vi "Hardware Discovery.vi"() -> ()   [LabVIEW 2020]
uses:
  subVIs/TypeDefs/rad_State Data.ctl
  subVIs/Targets/TypeDefs/rad_Targets Settings.ctl
  support/SubVIs/Target Information.ctl
  subVIs/Targets/TypeDefs/rad_Target Network Settings.ctl
  support/Controls/Discovery Settings.ctl
  support/Controls/Discovery Method Enum.ctl
  support/Controls/Important Paths.ctl
  subVIs/Util/Controls/Exit Button.ctl
  subVIs/Util/Controls/Refresh Button.ctl
  subVIs/Util/Controls/Configure Button.ctl
  subVIs/Util/Controls/Select All Button.ctl
  subVIs/Util/Controls/Add Target Button.ctl
  support/Controls/SetUp Btn.ctl
  subVIs/Util/FP Control/FP Control Functions.ctl
  <vilib>/Utility/miscctls.llb/LVRowAndColumnUnsignedTypeDef.ctl
  support/Message Queue/Enqueue Message (Single).vi
  <vilib>/nisyscfg/Close (System).vi
  support/Message Queue/Message Queue.lvlib
  <vilib>/nisyscfg/nisyscfg.lvlib
  <resource>/objmgr/nisysapi.rc
panel:
  in  "Set Up Target":T1
  in  "Exit":T2
  in  "Target List":i32[](listbox)=[0]
  in  "Refresh Targets":T3
  in  "Targets Settings":bool
  in  "Add Target":T4
  in  "Select All":T5
  in  "Configure Targets":T6
  in  "App Data":T7 {"Targets Information"."Primary NIC"."IP Address Request Mode" items=["Static"=1, "DHCP/Link-Local"=2, "Link-Local Only"=4, "DHCP Only"=8]}
  # "Detected Targets"
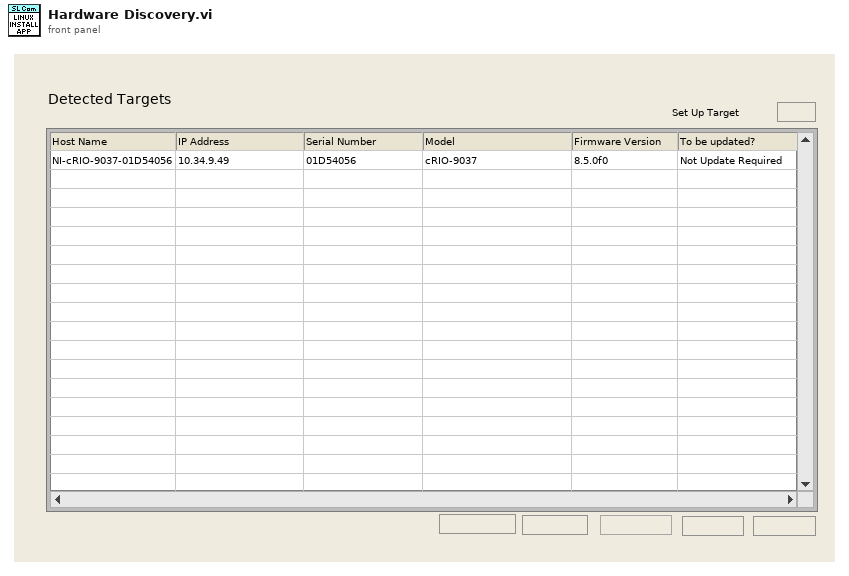
[diagram p1: front panel]
types:
  T1 = typedef "SetUp Btn.ctl" = bool
  T2 = typedef "Exit Button.ctl" = bool
  T3 = typedef "Refresh Button.ctl" = bool
  T4 = typedef "Add Target Button.ctl" = bool
  T5 = typedef "Select All Button.ctl" = bool
  T6 = typedef "Configure Button.ctl" = bool
  T7 = typedef "rad_State Data.ctl" = cluster{"Targets Settings":T8, "Targets Information":T9[], "Filtered Targets":i32[], "AppMode":string, "Configuration File Path":path, "Permissions":cluster{"Retrieve AppImgs":bool}, "User Added Targets":string[], "Discovery":T11, "Important Paths":T13}
  T8 = typedef "rad_Targets Settings.ctl" = cluster{"Target Types":string[], "Reduce Discovery Timeout":bool}
  T9 = typedef "Target Information.ctl" = cluster{"Hostname":string, "Serial number":string, "Product name":string, "Product code":i32, "System status":string, "Credential type":enum16{"None/Unlocked", "FTP Password", "NIAuth Credentials"}, "User added?":bool, "Primary NIC":T10}
  T10 = typedef "rad_Target Network Settings.ctl" = cluster{"MAC address":string, "IP Address Request Mode":i32, "IP address":string, "Subnet mask":string, "Gateway":string, "DNS server":string}
  T11 = typedef "Discovery Settings.ctl" = cluster{"Method":T12, "NotAsk":bool, "IPsFilePath":path}
  T12 = typedef "Discovery Method Enum.ctl" = enum32{"USB", "IPsFile", "AutoAll", "NotDiscover"}
  T13 = typedef "Important Paths.ctl" = cluster{"Linux Base Image":path, "Firmware Locations":path, "System Configuration Version":string}
  T14 = typedef "LVPoint32TypeDef.ctl" = cluster{"Horizontal":i32, "Vertical":i32}
  T15 = typedef "LVRowAndColumnTypeDef.ctl" = cluster{"Row":i32, "Column":i32}
  T16 = typedef "LVRowAndColumnUnsignedTypeDef.ctl" = cluster{"Row":u32, "Column":u32}
  T17 = enum8{"Enabled", "Disabled", "Disabled and Grayed Out"}
  T18 = typedef "FP Control Functions.ctl" = enum16{"Open", "Close", "Bring To Front", "Center"}
  T19 = enum32{"invalid app kind", "Development System", "Run Time System", "Student Edition", "Embedded LabVIEW", "Evaluation", "Custom"}
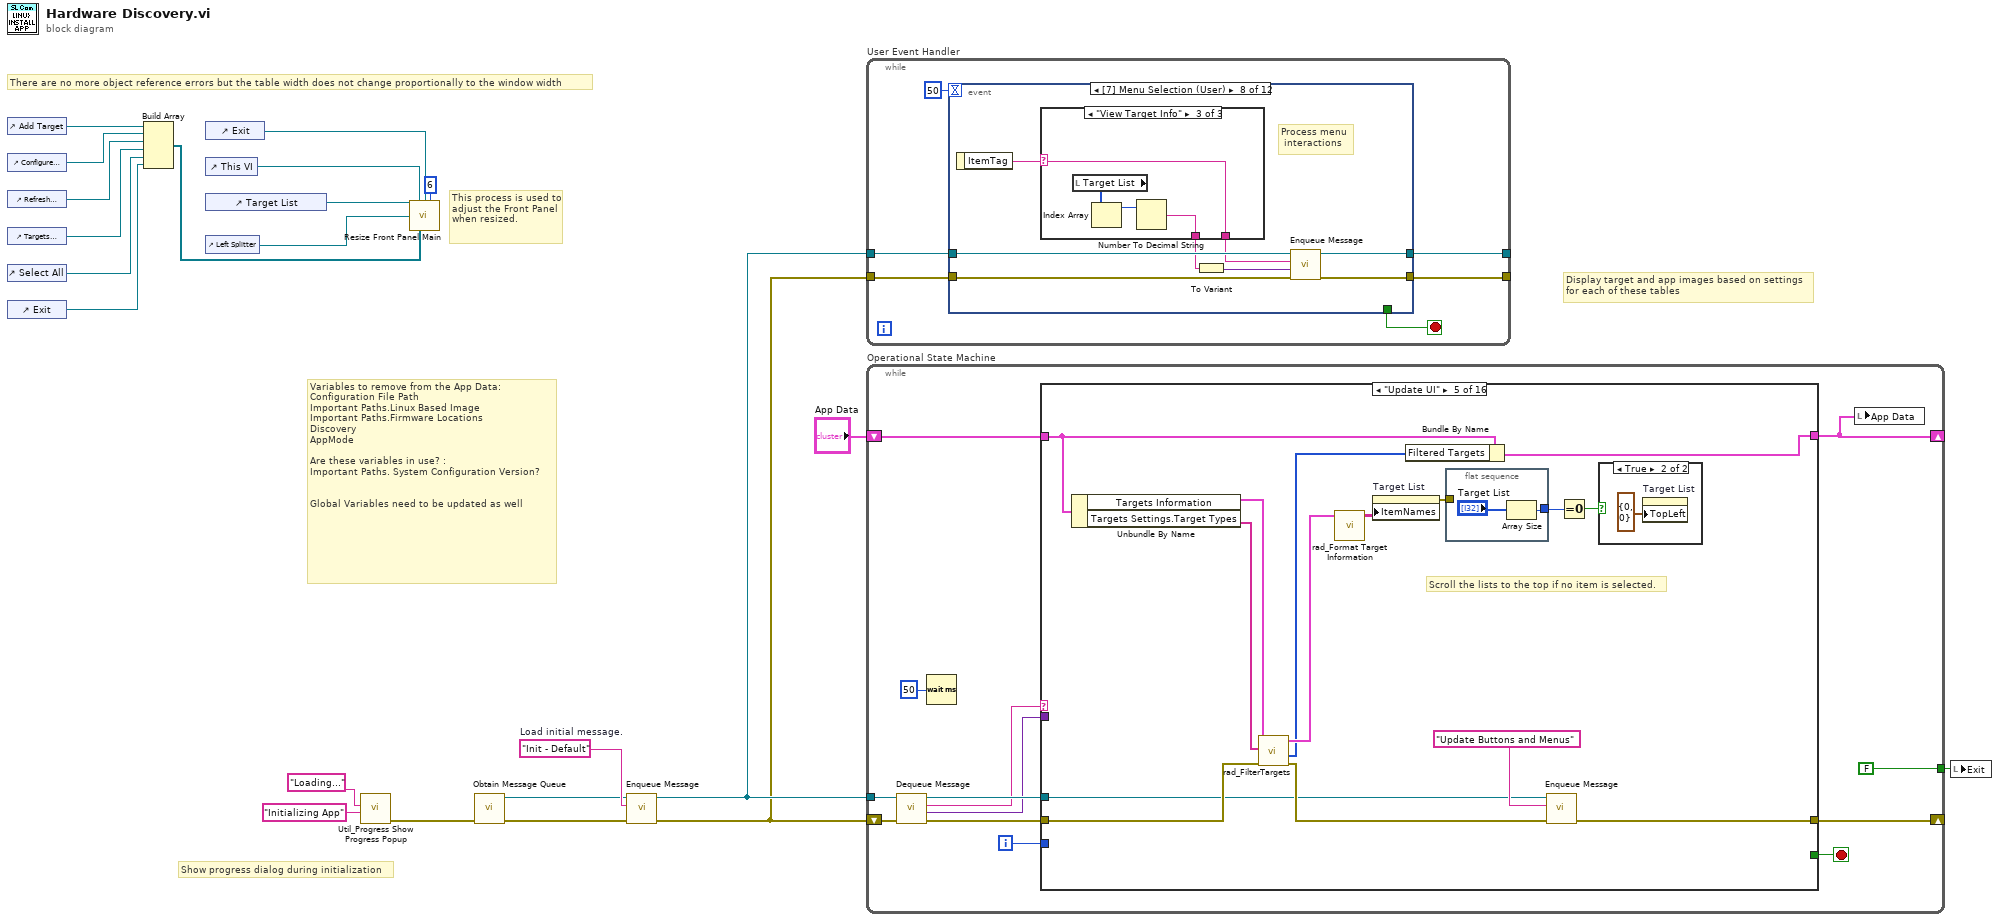
[diagram p0: block diagram]
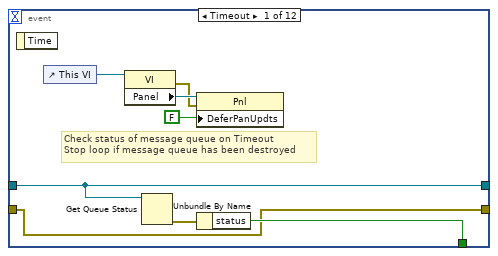
[diagram p2: hidden frame]
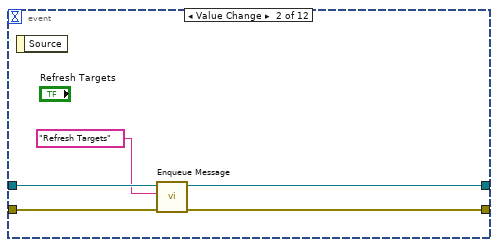
[diagram p3: hidden frame]
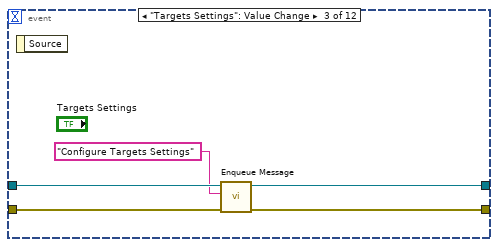
[diagram p4: hidden frame]
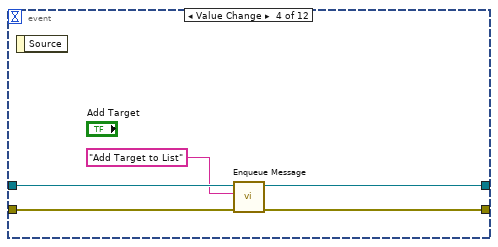
[diagram p5: hidden frame]
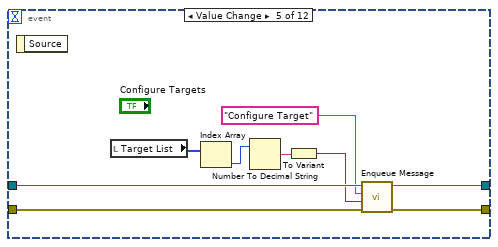
[diagram p6: hidden frame]
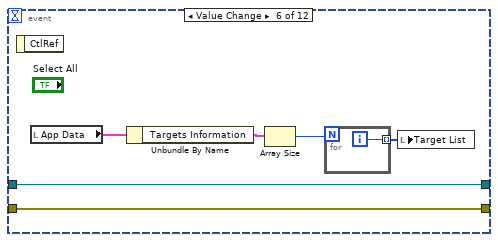
[diagram p7: hidden frame]
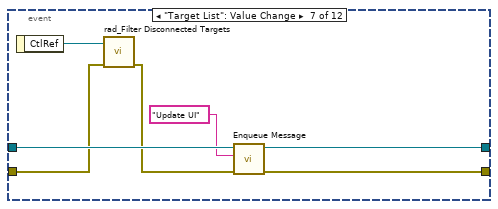
[diagram p8: hidden frame]
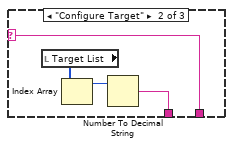
[diagram p10: hidden frame]
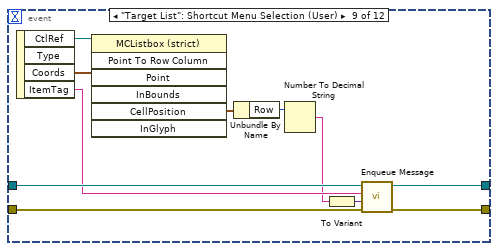
[diagram p11: hidden frame]
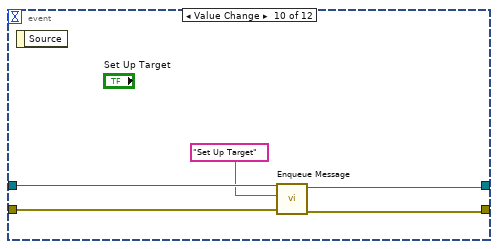
[diagram p12: hidden frame]
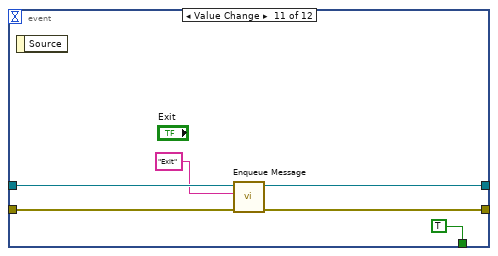
[diagram p13: hidden frame]
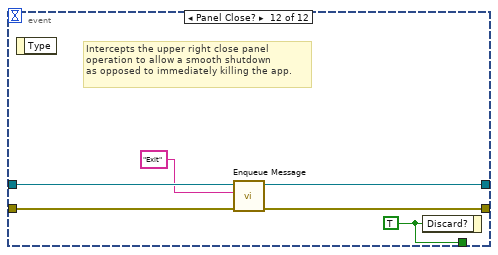
[diagram p14: hidden frame]
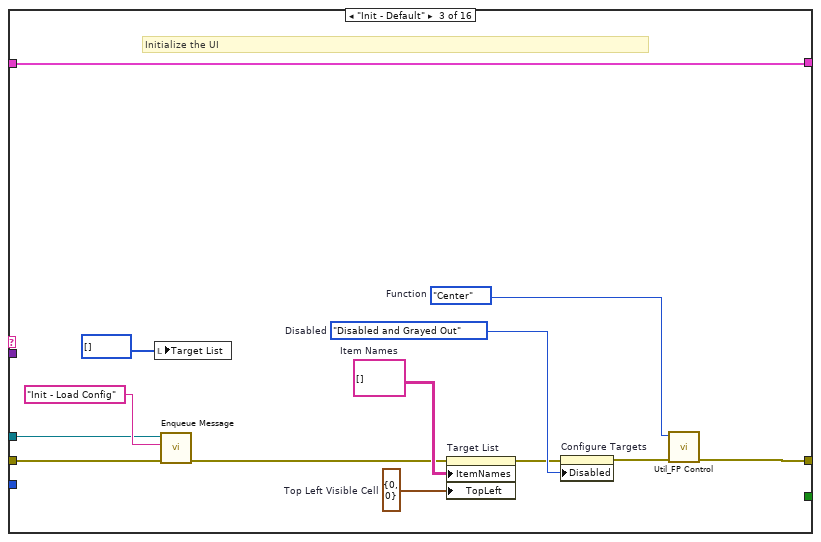
[diagram p17: hidden frame]
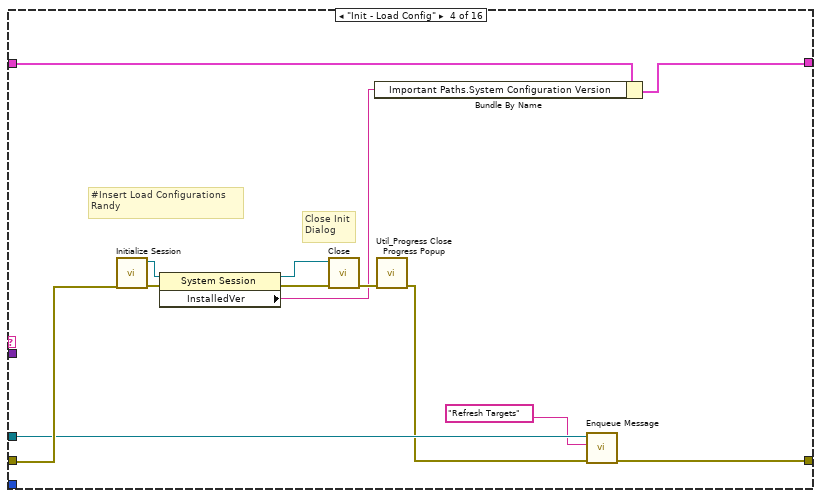
[diagram p18: hidden frame]
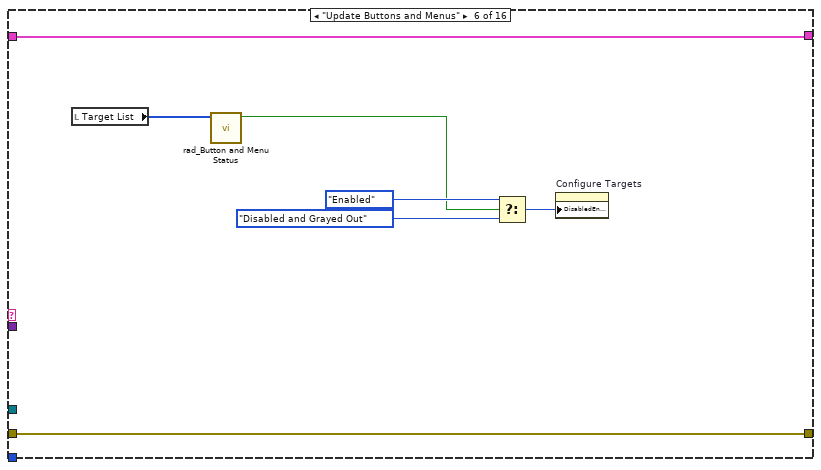
[diagram p20: hidden frame]
diagram:
  w8 = "Init - Default"  # Load initial message.
  # "Variables to remove from the App Data:\nConfiguration File Path\nImportant Paths.Linux Based Image\nImportant Paths.Firmware Locations\nDiscovery\nAppMode\n\nAre these variables in use? :\nImportant Paths. System Configuration Version?\n\n\nGlobal Variables need to be updated as well"
  # "There are no more object reference errors but the table width does not change proportionally to the window width"
  # "Display target and app images based on settings\nfor each of these tables"
  # "Show progress dialog during initialization"
  # "This process is used to adjust the Front Panel when resized."
  n1 = control-ref of="Add Target"() -> (w17:refnum<vi>)
  n2 = control-ref of="Configure Targets"() -> (w16:refnum<vi>)
  n3 = control-ref of="Refresh Targets"() -> (w15:refnum<vi>)
  n4 = control-ref of="Targets Settings"() -> (w14:refnum<vi>)
  n5 = control-ref of="Select All"() -> (w13:refnum<vi>)
  n6 = control-ref of="Exit"() -> (w3:refnum<vi>)
  n7 = Build Array(w17, w16, w15, w14, w13, w3) -> (w12:refnum<vi>[])
  n8 = control-ref of="Exit"() -> (w21:refnum<vi>)
  n9 = control-ref of="This VI"() -> (w20:refnum<vi>)
  n10 = control-ref of="Target List"() -> (w19:refnum<vi>)
  n11 = control-ref of="Left Splitter"() -> (w18:refnum<vi>)
  n12 = call "Util_Progress Show Progress Popup.vi"("Title"="Initializing App", "Message"="Loading...") -> ("error out"=w10:errorcluster)  [unwired: 2 in, 7 out]
  n13 = call "Resize Front Panel Main.vi"("Left Listbox"=w19, "Top Level VI"=w20, "Stop"=w21, "Number of Columns"=6, "Left Splitter"=w18, "Left Pane Items"=w12) -> ()  [unwired: 9 in, 1 out]
  n14 = call "Obtain Message Queue.vi"("error in (no error)"=w10) -> ("error out"=w9:errorcluster, "Message Queue"=w7:refnum<queue>)  [unwired: 9 in]
  n15 = call-poly "Enqueue Message.vi"("error in (no error)"=w9, "Message"=w8, "Message Queue"=w7) -> ("error out"=w5:errorcluster, "dup Message Queue"=w6:refnum<queue>)  [unwired: 7 in]
  n16 = while "User Event Handler" {
    tunnel: w6 -> [w26]
    tunnel: [w25] -> _
    tunnel: w5 -> [w24]
    tunnel: [w23] -> _
    stop <- w27 stop-if-true
    n17 = event shown="[7] Menu Selection (User)" {
      selector: _ -> [_ _ _ _ _ _ _ _ _ _ _ _]
      dyn-events: _ -> [_ _ _ _ _ _ _ _ _ _ _ _]
      timeout: 50 -> [_ _ _ _ _ _ _ _ _ _ _ _]
      tunnel: [w34 _ _ _ _ _ _ _ _ _ TRUE ("Discard?") w119] -> w27
      tunnel: w26 -> [w36 w41 w44 w49 w56 w62 w72 w79 w96 w107 w110 w116]
      tunnel: [w36 w40 w43 w48 w55 w62 w71 w78 w95 w105 w109 w115] -> w25
      tunnel: w24 -> [w29 w39 w46 w51 w58 w61 w68 w81 w98 w106 w112 w118]
      tunnel: [w29 w38 w45 w50 w57 w61 w73 w80 w97 w104 w111 w117] -> w23
      event Timeout {
        # "Check status of message queue on Timeout\nStop loop if message queue has been destroyed"
        n18 = event-data() -> ()  [unwired: 2 out]
        n19 = control-ref of="This VI"() -> (w30:refnum<vi>)
        n20 = property class="VI"(reference=w30) -> (error out=w31:errorcluster, "Panel"=w33:refnum<vi>)  [unwired: 1 in, 1 out]
        n21 = Get Queue Status(queue=w36) -> (error out=w35:errorcluster)  [unwired: 1 in, 8 out]
        n22 = property class="Pnl"(reference=w33, error in=w31, "DeferPanUpdts"=FALSE ("Defer Panel Updates")) -> ()  [unwired: 2 out]
        n23 = Unbundle By Name(w35) -> ("status"=w34:bool)
      }
      event Value Change {
        n24 = event-data() -> ()  [unwired: 2 out]
        n25 = call-poly "Enqueue Message.vi"("error in (no error)"=w39, "Message"="Refresh Targets", "Message Queue"=w41) -> ("error out"=w38:errorcluster, "dup Message Queue"=w40:refnum<queue>)  [unwired: 7 in]
      }
      event "Targets Settings": Value Change {
        n26 = event-data() -> ()  [unwired: 2 out]
        n27 = call-poly "Enqueue Message.vi"("error in (no error)"=w46, "Message"="Configure Targets Settings", "Message Queue"=w44) -> ("error out"=w45:errorcluster, "dup Message Queue"=w43:refnum<queue>)  [unwired: 7 in]
      }
      event Value Change {
        n28 = event-data() -> ()  [unwired: 2 out]
        n29 = call-poly "Enqueue Message.vi"("error in (no error)"=w51, "Message"="Add Target to List" ("Message Name"), "Message Queue"=w49) -> ("error out"=w50:errorcluster, "dup Message Queue"=w48:refnum<queue>)  [unwired: 7 in]
      }
      event Value Change {
        n30 = event-data() -> ()  [unwired: 2 out]
        n31 = local read "Target List"() -> (w59:i32[])
        n32 = Index Array(array=w59) -> (element=w60:i32)  [unwired: 1 in]
        n33 = Number To Decimal String(number=w60) -> (decimal integer string=w54:string)  [unwired: 1 out]
        n34 = To Variant(anything=w54) -> (Variant=w53:variant)
        n35 = call-poly "Enqueue Message.vi"("error in (no error)"=w58, "Message Data"=w53, "Message"="Configure Target", "Message Queue"=w56) -> ("error out"=w57:errorcluster, "dup Message Queue"=w55:refnum<queue>)  [unwired: 6 in]
      }
      event Value Change {
        n36 = event-data() -> ()  [unwired: 2 out]
        n37 = local read "App Data"() -> (w65:T7)
        n38 = Unbundle By Name(w65) -> ("Targets Information"=w64:T9[])
        n39 = Array Size(array=w64) -> (size(s)=w63:i32)
        n40 = for {
          N: w63 -> [_]
          tunnel: [w67] -> w66 mode=indexing
          i -> [w67]
        }
        n41 = local write "Target List"(w66) -> ()
      }
      event "Target List": Value Change {
        n42 = event-data() -> ("CtlRef"=w74:refnum<vi>)  [unwired: 1 out]
        n43 = call "rad_Filter Disconnected Targets.vi"("error in (no error)"=w68, "Target List Ref"=w74) -> ("error out"=w69:errorcluster)  [unwired: 9 in]
        n44 = call-poly "Enqueue Message.vi"("error in (no error)"=w69, "Message"="Update UI", "Message Queue"=w72) -> ("error out"=w73:errorcluster, "dup Message Queue"=w71:refnum<queue>)  [unwired: 7 in]
      }
      event Menu Selection (User) {
        # "Process menu\n interactions"
        n45 = event-data() -> ("ItemTag"=w82:string)  [unwired: 1 out]
        n46 = case shown="\"View Target Info\"" w82 {
          selector: w82 -> [w83 w85 w89]
          tunnel: [w83 w85 w89] -> w77
          tunnel: [_ w84 w88] -> w76
          frame Default {
          }
          frame "Configure Target" {
            n47 = local read "Target List"() -> (w87:i32[])
            n48 = Index Array(array=w87) -> (element=w86:i32)  [unwired: 1 in]
            n49 = Number To Decimal String(number=w86) -> (decimal integer string=w84:string)  [unwired: 1 out]
          }
          frame "View Target Info" {
            n50 = local read "Target List"() -> (w91:i32[])
            n51 = Index Array(array=w91) -> (element=w90:i32)  [unwired: 1 in]
            n52 = Number To Decimal String(number=w90) -> (decimal integer string=w88:string)  [unwired: 1 out]
          }
        }
        n53 = To Variant(anything=w76) -> (Variant=w75:variant)
        n54 = call-poly "Enqueue Message.vi"("error in (no error)"=w81, "Message Data"=w75, "Message"=w77, "Message Queue"=w79) -> ("error out"=w80:errorcluster, "dup Message Queue"=w78:refnum<queue>)  [unwired: 6 in]
      }
      event "Target List": Shortcut Menu Selection (User) {
        n55 = event-data() -> ("CtlRef"=w100:refnum<vi>, "Coords"=w99:T14, "ItemTag"=w94:string)  [unwired: 2 out]
        n56 = invoke class="MCListbox (strict)" method="Point To Row Column"(reference=w100, "Point"=w99) -> ("CellPosition"=w102:T15)  [unwired: 5 in, 6 out]
        n57 = Unbundle By Name(w102) -> ("Row"=w101:i32)
        n58 = Number To Decimal String(number=w101) -> (decimal integer string=w93:string)  [unwired: 1 out]
        n59 = To Variant(anything=w93) -> (Variant=w92:variant)
        n60 = call-poly "Enqueue Message.vi"("error in (no error)"=w98, "Message Data"=w92, "Message"=w94, "Message Queue"=w96) -> ("error out"=w97:errorcluster, "dup Message Queue"=w95:refnum<queue>)  [unwired: 6 in]
      }
      event Value Change {
        n61 = event-data() -> ()  [unwired: 2 out]
        n62 = call-poly "Enqueue Message.vi"("error in (no error)"=w106, "Message"="Set Up Target", "Message Queue"=w107) -> ("error out"=w104:errorcluster, "dup Message Queue"=w105:refnum<queue>)  [unwired: 7 in]
      }
      event Value Change {
        n63 = event-data() -> ()  [unwired: 2 out]
        n64 = call-poly "Enqueue Message.vi"("error in (no error)"=w112, "Message"="Exit", "Message Queue"=w110) -> ("error out"=w111:errorcluster, "dup Message Queue"=w109:refnum<queue>)  [unwired: 7 in]
      }
      event Panel Close? {
        w119 = TRUE ("Discard?")
        # "Intercepts the upper right close panel\noperation to allow a smooth shutdown\nas opposed to immediately killing the app."
        n65 = event-data() -> ()  [unwired: 2 out]
        n66 = call-poly "Enqueue Message.vi"("error in (no error)"=w118, "Message"="Exit", "Message Queue"=w116) -> ("error out"=w117:errorcluster, "dup Message Queue"=w115:refnum<queue>)  [unwired: 7 in]
        n67 = event-data("Discard?"=w119) -> ()  [unwired: 1 in, 1 out]
      }
    }
  }
  n68 = while "Operational State Machine" {
    shift-left: w5 -> [w127]
    shift-right: [w131] -> _
    tunnel: w6 -> [w125]
    tunnel: [T2 FALSE ("Exit")] -> w11
    shift-right: [w120] -> _
    shift-left: "App Data" -> [w121]
    i -> [w132]
    stop <- w129 stop-if-true
    n69 = call "Dequeue Message.vi"("error in (no error)"=w127, "Message Queue"=w125) -> ("error out"=w126:errorcluster, "Message Data"=w122:variant, "Message"=w123:string, "dup Message Queue"=w124:refnum<queue>)  [unwired: 6 in]
    n70 = Wait (ms)(milliseconds to wait=u32 50) -> ()  [unwired: 1 out]
    n71 = case shown="\"Update UI\"" w123 {
      tunnel: [w133 w135 w137 w153 w168 w187 w188 w192 w203 w207 w225 w251 w265 w281 w293 w303] -> w120
      tunnel: w124 -> [_ _ w142 w155 w163 _ _ _ _ w209 w228 w253 w271 _ _ _]
      tunnel: w126 -> [w134 w136 w145 w157 w167 w181 w190 w193 w204 w215 w230 w249 w270 w284 w292 w302]
      tunnel: w132 -> [_ _ _ _ _ _ _ _ _ _ _ _ _ _ _ _]
      tunnel: w122 -> [_ _ _ _ _ _ _ _ _ _ _ w250 _ w279 _ _]
      tunnel: [w134 w136 w139 w158 w165 w181 errorcluster {"status"=FALSE, "code"=0, "source"=""} ("error out") w195 w204 w210 w229 w255 w267 w280 w292 w297] -> w131
      tunnel: [_ _ _ _ _ _ _ TRUE _ _ _ _ _ _ _ _] -> w129
      tunnel: w121 -> [w133 w135 w137 w151 w169 w187 w188 w192 w203 w206 w226 w252 w264 w281 w293 w303]
      frame "Missing Message Handler", Default {
      }
      frame "**** General Application Messages ****" {
      }
      frame "Init - Default" {
        w141 = T17."Disabled and Grayed Out"  # Disabled
        w146 = T16 {"Row"=0, "Column"=0}  # Top Left Visible Cell
        w147 = FP_Control_Functions."Center"  # Function
        w148 = string[][] []  # Item Names
        # "Initialize the UI"
        n72 = local write "Target List"(i32[] [] ("Target List")) -> ()
        n73 = call-poly "Enqueue Message.vi"("error in (no error)"=w145, "Message"="Init - Load Config", "Message Queue"=w142) -> ("error out"=w144:errorcluster)  [unwired: 7 in, 1 out]
        n74 = property on="Target List" class="MCListbox (strict)"(error in=w144, "ItemNames"=w148, "TopLeft"=w146) -> (error out=w140:errorcluster)  [unwired: 1 in, 1 out]
        n75 = property on="Configure Targets" class="Bool"(error in=w140, "Disabled"=w141) -> (error out=w138:errorcluster)  [unwired: 1 in, 1 out]
        n76 = call "Util_FP Control.vi"("error in (no error)"=w138, "Function"=w147) -> ("error out"=w139:errorcluster)  [unwired: 9 in]
      }
      frame "Init - Load Config" {
        # "#Insert Load Configurations\nRandy"
        # "Close Init\nDialog"
        n77 = call <vilib>:"Initialize Session.vi"("error in (no error)"=w157) -> ("error out"=w160:errorcluster, "Session out"=w161:refnum<k21>)  [unwired: 9 in]
        n78 = property class="System Session"(reference=w161, error in=w160) -> (reference out=w162:refnum<k21>, error out=w159:errorcluster, "InstalledVer"=w152:string)
        n79 = call-poly <vilib>:"Close.vi"("error in (no error)"=w159, "Session in"=w162) -> ("error out"=w156:errorcluster)  [unwired: 9 in]
        n80 = Bundle By Name(cluster=w151, "Important Paths.System Configuration Version"=w152) -> (w153:T7)
        n81 = call "Util_Progress Close Progress Popup.vi"("error in (no error)"=w156) -> ("error out"=w154:errorcluster)  [unwired: 2 in, 8 out]
        n82 = call-poly "Enqueue Message.vi"("error in (no error)"=w154, "Message"="Refresh Targets", "Message Queue"=w155) -> ("error out"=w158:errorcluster)  [unwired: 7 in, 1 out]
      }
      frame "Update UI" {
        # "Scroll the lists to the top if no item is selected."
        n83 = Unbundle By Name(w169) -> ("Targets Information"=w177:T9[], "Targets Settings.Target Types"=w173:string[])
        n84 = call "rad_FilterTargets.vi"("error in (no error)"=w167, "Target Types"=w173, "Targets Information"=w177) -> ("error out"=w166:errorcluster, "Filtered Targets"=w175:i32[], "Targets Information"=w176:T9[])  [unwired: 6 out]
        n85 = call "rad_Format Target Information.vi"("Targets Information"=w176) -> ("Targets Information"=w174:string[][])  [unwired: 10 out]
        n86 = property on="Target List" class="MCListbox (strict)"("ItemNames"=w174) -> (error out=w172:errorcluster)  [unwired: 2 in, 1 out]
        n87 = Bundle By Name(cluster=w169, "Filtered Targets"=w175) -> (w168:T7)
        n88 = flat-sequence {
          tunnel: w172 -> [_]
          tunnel: [w179] -> w171
          frame #0 {
            n89 = Array Size(array="Target List") -> (size(s)=w179:i32)
          }
        }
        n90 = call-poly "Enqueue Message.vi"("error in (no error)"=w166, "Message"="Update Buttons and Menus" ("Message Name"), "Message Queue"=w163) -> ("error out"=w165:errorcluster)  [unwired: 7 in, 1 out]
        n91 = Equal To 0?(x=w171) -> (x = 0?=w170:bool)
        n92 = case shown="True" w170 {
          frame False {
          }
          frame True {
            n93 = property on="Target List" class="MCListbox (strict)"("TopLeft"=T16 {"Row"=0, "Column"=0} ("Top Left Visible Cell")) -> ()  [unwired: 2 in, 2 out]
          }
        }
      }
      frame "Update Buttons and Menus" {
        n94 = local read "Target List"() -> (w186:i32[])
        n95 = call "rad_Button and Menu Status.vi"("Target List"=w186) -> ("Configure Target"=w183:bool)  [unwired: 9 in, 1 out]
        n96 = Select(t=T17."Enabled" ("Disabled"), s=w183, f=T17."Disabled and Grayed Out" ("Disabled")) -> (s? t:f=w182:T17)
        n97 = property on="Configure Targets" class="Bool"("DisabledEnum"=w182) -> ()  [unwired: 2 in, 2 out]
      }
      frame "Error" {
        # "Display run-time error message\nAdd code to log error if desired"
        n98 = disable-structure shown="TARGET_TYPE==Windows" {
          disable-tunnel: w190 -> [w191 _]
          frame condition #0 (active) {
            n99 = call <vilib>:"Simple Error Handler.vi"("error in (no error)"=w191) -> ()  [unwired: 1 in, 8 out]
          }
          frame condition #1 {
          }
        }
      }
      frame "Exit" {
        # "#Inser Write Configuration File\nRandy"
        # "Close the front panel if the application is running as an EXE"
        n100 = Open Application Reference() -> (0:w198:errorcluster, 3:w199:refnum<vi>)  [unwired: 4 in]
        n101 = property class="App"(reference=w199, error in=w198) -> ("App.Kind"=w197:T19)  [unwired: 2 out]
        n102 = case shown="\"Run Time System\"" w197 {
          frame Default {
          }
          frame "Run Time System" {
            # "Close FP in EXE"
            n103 = Current VI's Path() -> (path=w202:path)
            n104 = Open VI Reference(vi path=w202) -> (vi reference=w201:refnum<vi>, error out=w200:errorcluster)  [unwired: 5 in]
            n105 = invoke class="VI" method="FP.Close"(reference=w201, error in=w200) -> ()  [unwired: 1 in, 3 out]
          }
        }
        n106 = property on="Exit" class="Bool (strict)"(error in=w193, "Val(Sgnl)"=TRUE) -> (error out=w195:errorcluster)  [unwired: 1 in, 1 out]
      }
      frame "**** Target Messages ****" {
      }
      frame "Refresh Targets" {
        # "Refresh list of RT targets on the local subnet.\nShow progress dialog during this process."
        n107 = Unbundle By Name(w206) -> ("Targets Settings.Reduce Discovery Timeout"=w213:bool, "User Added Targets"=w221:string[], "Targets Settings.Target Types"=w212:string[])
        n108 = call "Util_Progress Show Progress Popup.vi"("error in (no error)"=w215, "Title"="Discovering Targets", "Message"="Refreshing target list...") -> ("error out"=w214:errorcluster)  [unwired: 1 in, 7 out]
        n109 = Search 1D Array(1D array=w212, element="User Targets Only") -> (index of element=w218:i32)  [unwired: 1 in]
        n110 = Not Equal?(x=w218, y=-1) -> (x != y?=w216:bool)
        n111 = call "rad_Refresh Target Information.vi"("Reduce Discovery Timeout"=w213, "error in (no error)"=w214, "User Added Targets Only"=w216, "User Added Targets"=w221) -> ("error out"=w211:errorcluster, "Targets Information"=w220:T9[])  [unwired: 6 in]
        n112 = call "Util_Progress Close Progress Popup.vi"("error in (no error)"=w211) -> ("error out"=w205:errorcluster)  [unwired: 2 in, 8 out]
        n113 = Bundle By Name(cluster=w206, "Targets Information"=w220) -> (w207:T7)
        n114 = call-poly "Enqueue Message.vi"("error in (no error)"=w205, "Message"="Update UI", "Message Queue"=w209) -> ("error out"=w210:errorcluster)  [unwired: 7 in, 1 out]
      }
      frame "Add Target to List" {
        n115 = Unbundle By Name(w226) -> ("User Added Targets"=w232:string[])
        n116 = call "rad_Add Target By IP Dialog.vi"() -> ("Canceled?"=w227:bool, "IP Address"=w231:string)  [unwired: 10 in]
        n117 = case shown="False" w227 {
          tunnel: w232 -> [w240 w245]
          tunnel: w231 -> [w239 _]
          tunnel: [w241 w245] -> w224
          frame False {
            n118 = Search 1D Array(1D array=w240, element=w239) -> (index of element=w244:i32)  [unwired: 1 in]
            n119 = Build Array (concatenate)(w240, w239) -> (w238:string[])
            n120 = Not Equal?(x=w244, y=-1) -> (x != y?=w242:bool)
            n121 = Select(t=w240, s=w242, f=w238) -> (s? t:f=w241:string[])
          }
          frame True {
          }
        }
        n122 = case shown="False" w227 {
          tunnel: w230 -> [w236 w237]
          tunnel: [w235 w237] -> w229
          tunnel: w228 -> [w233 _]
          frame False {
            n123 = call-poly "Enqueue Message.vi"("error in (no error)"=w236, "Message"="Refresh Targets" ("Message Name"), "Message Queue"=w233) -> ("error out"=w235:errorcluster)  [unwired: 7 in, 1 out]
          }
          frame True {
          }
        }
        n124 = Bundle By Name(cluster=w226, "User Added Targets"=w224) -> (w225:T7)
      }
      frame "Configure Target" {
        # "Update network settings/configuration of the selected RT target"
        n125 = Variant To Data(error in=w249, type="", Variant=w250) -> (data=w246:string, error out=w248:errorcluster)
        n126 = Unbundle By Name(w252) -> ("Targets Information"=w260:T9[], "Filtered Targets"=w263:i32[])
        n127 = Decimal String To Number(string=w246) -> (number=w262:i32)  [unwired: 3 out]
        n128 = Index Array(array=w263, index=w262) -> (element=w258:i32)
        n129 = Index Array(array=w260, index=w258) -> (element=w261:T9)
        n130 = call "rad_Configure Target Dialog.vi"("Error In"=w248, "Target Information in"=w261) -> ("Error Out"=w256:errorcluster, "Target Information out"=w259:T9)  [unwired: 8 out]
        n131 = Replace Array Subset(array=w260, new element=w259, index=w258) -> (w257:T9[])
        n132 = call <vilib>:"General Error Handler.vi"("error in (no error)"=w256) -> ()  [unwired: 10 in, 5 out]
        n133 = Bundle By Name(cluster=w252, "Targets Information"=w257) -> (w251:T7)
        n134 = call-poly "Enqueue Message.vi"("error in (no error)"=w248, "Message"="Update UI", "Message Queue"=w253) -> ("error out"=w255:errorcluster)  [unwired: 7 in, 1 out]
      }
      frame "Configure Targets Settings" {
        # "Configures the Global Timeout"
        n135 = Unbundle By Name(w264) -> ("Targets Settings"=w268:T8)
        n136 = call "rad_Configure Targets Settings Dialog.vi"("Targets Settings"=w268) -> ("Targets Settings"=w269:T8)  [unwired: 10 out]
        n137 = Equal?(x=w269, y=w268) -> (x = y?=w266:bool)
        n138 = Bundle By Name(cluster=w264, "Targets Settings"=w269) -> (w265:T7)
        n139 = case shown="False" w266 {
          tunnel: w271 -> [w273 _]
          tunnel: w270 -> [w275 w276]
          tunnel: [w274 w276] -> w267
          frame False {
            n140 = call-poly "Enqueue Message.vi"("error in (no error)"=w275, "Message"="Update UI", "Message Queue"=w273) -> ("error out"=w274:errorcluster)  [unwired: 7 in, 1 out]
          }
          frame True {
          }
        }
      }
      frame "View Target Info" {
        # "Display additional information about \nthe selected RT target in a popup window"
        n141 = Variant To Data(error in=w284, type="", Variant=w279) -> (data=w278:string, error out=w280:errorcluster)
        n142 = Unbundle By Name(w281) -> ("Targets Information"=w289:T9[], "Filtered Targets"=w288:i32[])
        n143 = Decimal String To Number(string=w278) -> (number=w287:i32)  [unwired: 3 out]
        n144 = Index Array(array=w288, index=w287) -> (element=w286:i32)
        n145 = Index Array(array=w289, index=w286) -> (element=w282:T9)
        n146 = call "rad_Get Target Info (IP).vi"("error in (no error)"=w280, "Target settings in"=w282) -> ("error out"=w283:errorcluster, "Target settings out"=w285:T9)  [unwired: 8 in]
        n147 = case shown="No Error" w283 {
          selector: w283 -> [_ w291]
          tunnel: w285 -> [w290 _]
          frame No Error {
            n148 = call "rad_Target Info Dialog.vi"("Target Information"=w290) -> ()  [unwired: 11 out]
          }
          frame Error {
            n149 = call <vilib>:"General Error Handler.vi"("error in (no error)"=w291) -> ()  [unwired: 10 in, 5 out]
          }
        }
      }
      frame "*** SW Installation Message ****" {
      }
      frame "Set Up Target" {
        # "Filters selected targets"
        # "Updates the device's firmware if its version is lower than 7 and applies the\nlatest image found in the local system."
        n150 = call "Util_Progress Show Progress Popup.vi"("error in (no error)"=w302, "Title"="Hardware Set Up", "Message"="Setting up the targets") -> ("error out"=w301:errorcluster)  [unwired: 1 in, 7 out]
        n151 = Unbundle By Name(w303) -> ("Targets Information"=w295:T9[], "Filtered Targets"=w296:i32[])
        n152 = for {
          tunnel: w296 -> [w305] mode=indexing
          tunnel: w295 -> [w306]
          tunnel: [w304] -> w294 mode=indexing
          n153 = Index Array(array=w306, index=w305) -> (element=w304:T9)
        }
        n154 = for {
          tunnel: w301 -> [w310]
          tunnel: [w308] -> w298
          tunnel: w294 -> [w307] mode=indexing
          n155 = call "Apply Firmware.vi"("error in"=w310, "Target information"=w307) -> ("error out"=w309:errorcluster)  [unwired: 7 in, 2 out]
          n156 = call "Apply System Image.vi"("error in"=w309, "Target information"=w307) -> ("error out"=w308:errorcluster)  [unwired: 8 in, 1 out]
        }
        n157 = call "Util_Progress Close Progress Popup.vi"("error in (no error)"=w298) -> ("error out"=w297:errorcluster)  [unwired: 2 in, 8 out]
      }
    }
    n158 = local write "App Data"(w120) -> ()
  }
  n159 = local write "Exit"(w11) -> ()
